vi "Read DB File Path.vi"(8 "error in (no error)":errorcluster, 11 "SQLite configuration in":refnum<class "SQLite configuration.lvclass">) -> (0 "error out":errorcluster, 2 "DB File Path":string="/home/lvuser/sqlite.db", 3 "SQLite configuration out":refnum<class "SQLite configuration.lvclass">)   [LabVIEW 2014, in "SQLite configuration.lvclass"]
uses:
  SQLite configuration.lvclass
  SQLite configuration.lvclass/SQLite configuration.ctl
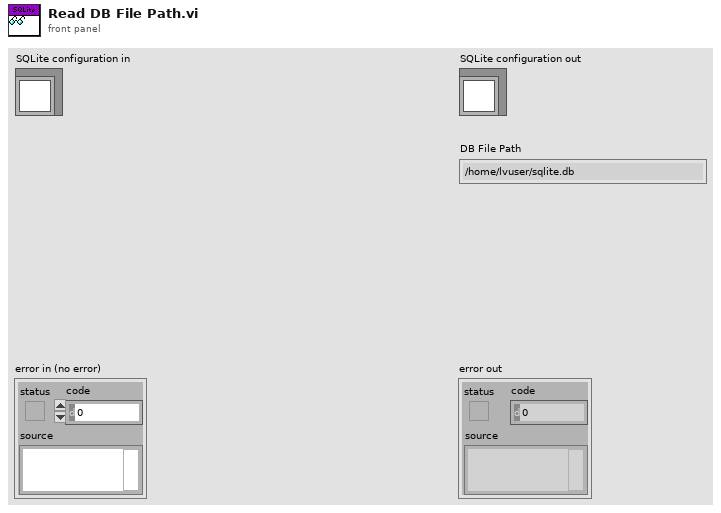
[diagram p1: front panel]
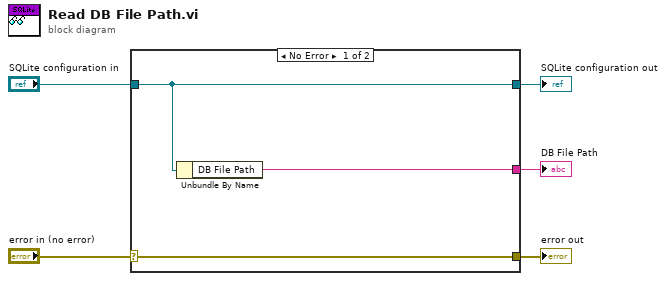
[diagram p0: block diagram]
diagram:
  n1 = case shown="No Error" "error in (no error)" {
    selector: "error in (no error)" -> [w8 w9]
    tunnel: [w8 w9] -> w4
    tunnel: [w7 w10] -> w2
    tunnel: "SQLite configuration in" -> [w7 w10]
    tunnel: [w6 _] -> w1
    frame No Error {
      n2 = Unbundle By Name(w7) -> ("DB File Path"=w6:string)
    }
    frame Error {
    }
  }
  "error out" <- w4
  "SQLite configuration out" <- w2
  "DB File Path" <- w1
